vi "Adjust Window Bounds for Desired Position.vi"(10 "Position":T2, 11 "Front Panel.WinBounds in":T1) -> (2 "Dimensions":cluster{"Width":i16, "Height":i16}, 3 "Front Panel.WinBounds out":T1)   [LabVIEW 2024, in "Dynamic Signal Acquisition (Interactive) UI.lvlib"]
uses:
  <vilib>/Utility/miscctls.llb/LVPositionTypeDef.ctl
  <vilib>/Utility/miscctls.llb/LVRectTypeDef.ctl
  Dynamic Signal Acquisition (Interactive) UI.lvlib
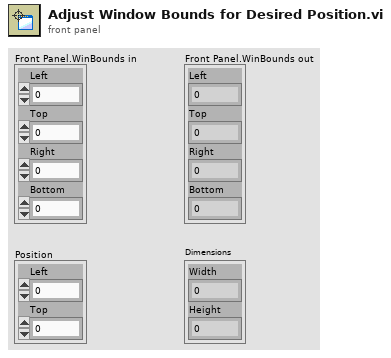
[diagram p1: front panel]
types:
  T1 = typedef "LVRectTypeDef.ctl" = cluster{"Left":i16, "Top":i16, "Right":i16, "Bottom":i16}
  T2 = typedef "LVPositionTypeDef.ctl" = cluster{"Left":i32, "Top":i32}
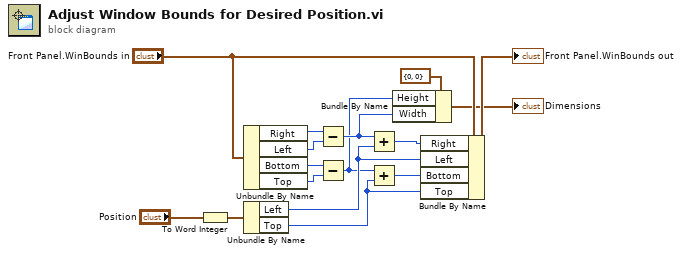
[diagram p0: block diagram]
diagram:
  n1 = To Word Integer(number="Position") -> (16bit integer=w14:cluster{"Left":i16, "Top":i16})
  n2 = Unbundle By Name("Front Panel.WinBounds in") -> ("Right"=w5:i16, "Left"=w6:i16, "Bottom"=w7:i16, "Top"=w8:i16)
  n3 = Unbundle By Name(w14) -> ("Left"=w11:i16, "Top"=w12:i16)
  n4 = Subtract(x=w5, y=w6) -> (x-y=w3:i16)
  n5 = Subtract(x=w7, y=w8) -> (x-y=w1:i16)
  n6 = Add(x=w3, y=w11) -> (x+y=w10:i16)
  n7 = Add(x=w1, y=w12) -> (x+y=w13:i16)
  n8 = Bundle By Name(cluster=cluster{"Width":i16, "Height":i16} {"Width"=0, "Height"=0} ("Dimensions"), "Height"=w1, "Width"=w3) -> (→"Dimensions":cluster{"Width":i16, "Height":i16})
  n9 = Bundle By Name(cluster="Front Panel.WinBounds in", "Right"=w10, "Left"=w11, "Bottom"=w13, "Top"=w12) -> (→"Front Panel.WinBounds out":T1)
